vi "test read UDP low.vi"() -> ()   [LabVIEW 2019]
uses:
  Controls/UDP - Command.ctl
  Controls/UDP - Event.ctl
  Controls/UDP - Status.ctl
  Controls/Communication - Write Data.ctl
panel:
  in  "Datalog":T1(ring)
  out "Channels":T2
  in  "local port":u16=4001
  in  "Zero":T3(ring)
  in  "remote port":u16=4001
  in  "address":string="192.168.88.50"
  out "Data System":T4
  in  "Data":T5
  out "Data ADC":T6
  out "PID Setting":T7
  out "Sensor Out":T8
  out "Test SP":T9
  out "Status":T10 items=["Stop", "Ramp Up", "Ramp Down", "Jog Up", "Jog Down", "PID Mode", "PID Ramp"]
  out "Event":T11 items=["Stop", "Running", "PID", "Up Limit", "Down Limit", "Load Limit"]
  out "CMD Decimal Form":u8[](array[numeric])
  out "CMD HEX Form":string
  out "x+y":i32
  in  "CMD":T12
  out "data out":string
  out "Numeric 2":u8
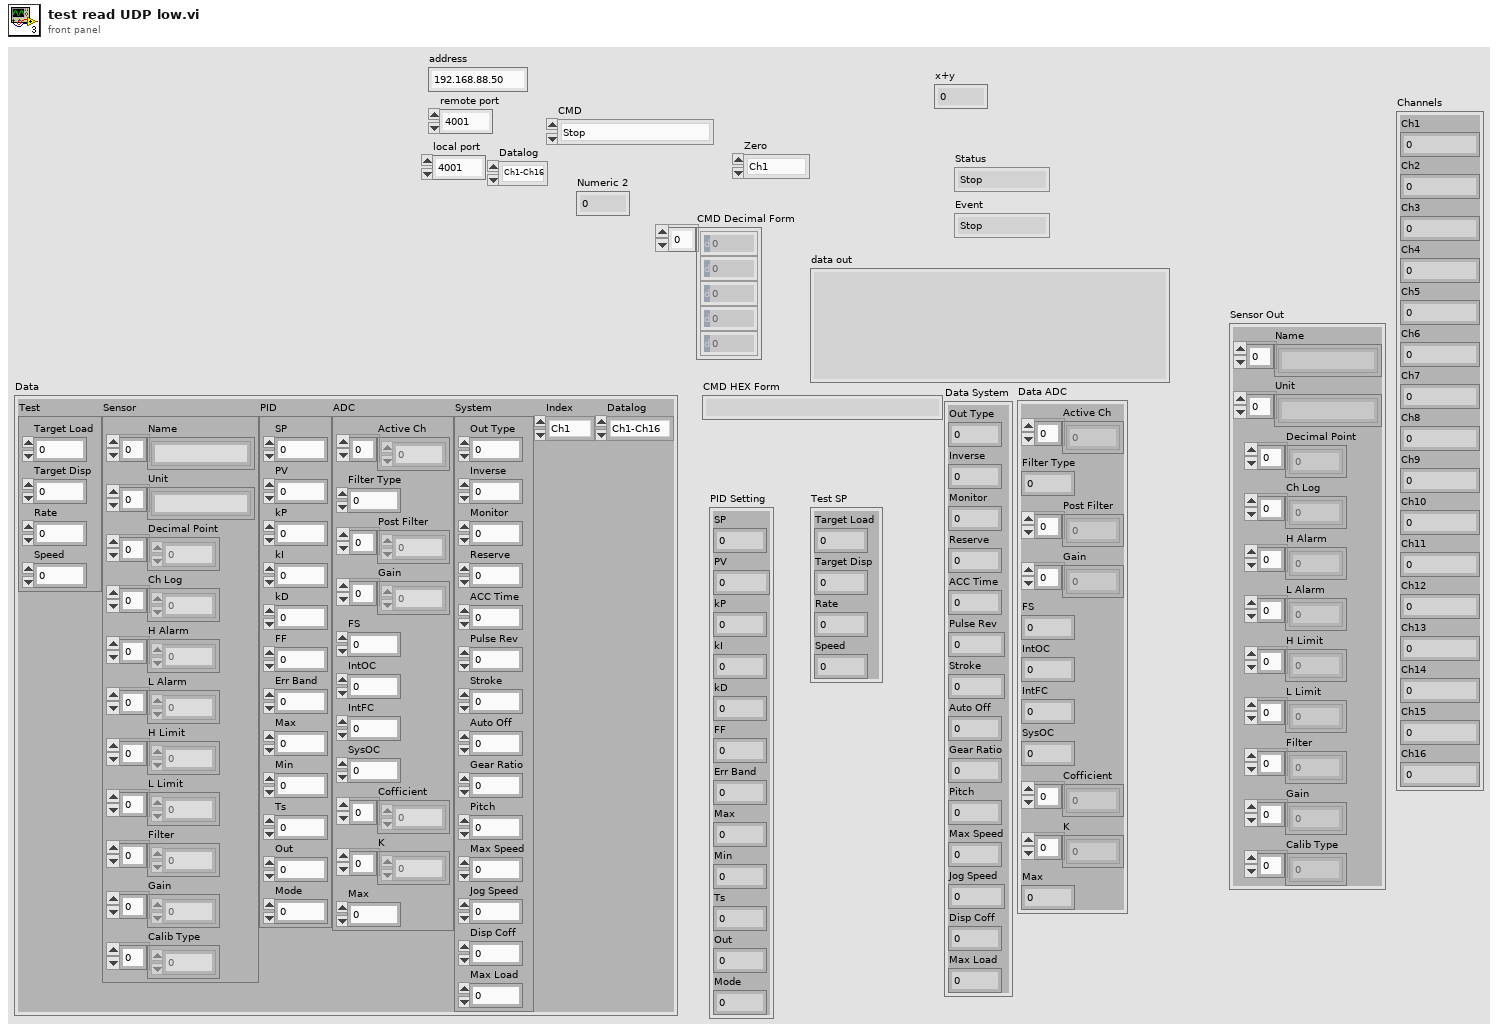
[diagram p1: front panel]
types:
  T1 = enum16{"Ch1-Ch16", "Ch17-Ch32", "Ch32-Ch48", "Ch49-Ch64", "Empty"}
  T2 = cluster{"Ch1":sgl, "Ch2":sgl, "Ch3":sgl, "Ch4":sgl, "Ch5":sgl, "Ch6":sgl, "Ch7":sgl, "Ch8":sgl, "Ch9":sgl, "Ch10":sgl, "Ch11":sgl, "Ch12":sgl, "Ch13":sgl, "Ch14":sgl, "Ch15":sgl, "Ch16":sgl}
  T3 = enum16{"Ch1", "Ch2", "Ch3", "Ch4", "Ch5", "Ch6", "Ch7", "Ch8", "Ch9", "Ch10", "Ch11", "Ch12", "Ch13", "Ch14", "Ch15", "Ch16"}
  T4 = cluster{"Out Type":u8, "Inverse":u8, "Monitor":u8, "Reserve":u8, "ACC Time":u32, "Pulse Rev":u32, "Stroke":u32, "Auto Off":u32, "Gear Ratio":sgl, "Pitch":sgl, "Max Speed":u32, "Jog Speed":u32, "Disp Coff":sgl, "Max Load":u32}
  T5 = typedef "Communication - Write Data.ctl" = cluster{"Test":cluster{"Target Load":sgl, "Target Disp":sgl, "Rate":sgl, "Speed":sgl}, "Sensor":cluster{"Name":string[], "Unit":string[], "Decimal Point":u8[], "Ch Log":u8[], "H Alarm":u8[], "L Alarm":u8[], "H Limit":sgl[], "L Limit":sgl[], "Filter":u8[], "Gain":u8[], "Calib Type":u32[]}, "PID":cluster{"SP":sgl, "PV":sgl, "kP":sgl, "kI":sgl, "kD":sgl, "FF":sgl, "Err Band":sgl, "Max":i32, "Min":i32, "Ts":u32, "Out":i32, "Mode":u8}, "ADC":cluster{"Active Ch":u8[], "Filter Type":u8, "Post Filter":u8[], "Gain":u8[], "FS":u16, "IntOC":u8, "IntFC":u8, "SysOC":u8, "Cofficient":dbl[], "K":dbl[], "Max":i32}, "System":cluster{"Out Type":u8, "Inverse":u8, "Monitor":u8, "Reserve":u8, "ACC Time":u32, "Pulse Rev":u32, "Stroke":u32, "Auto Off":u32, "Gear Ratio":sgl, "Pitch":sgl, "Max Speed":u32, "Jog Speed":u32, "Disp Coff":sgl, "Max Load":u32}, "Index":enum16{"Ch1", "Ch2", "Ch3", "Ch4", "Ch5", "Ch6", "Ch7", "Ch8", "Ch9", "Ch10", "Ch11", "Ch12", "Ch13", "Ch14", "Ch15", "Ch16"}, "Datalog":enum16{"Ch1-Ch16", "Ch17-Ch32", "Ch32-Ch48", "Ch49-Ch64", "Empty"}}
  T6 = cluster{"Active Ch":u8[], "Filter Type":u8, "Post Filter":u8[], "Gain":u8[], "FS":u16, "IntOC":u8, "IntFC":u8, "SysOC":u8, "Cofficient":dbl[], "K":dbl[], "Max":i32}
  T7 = cluster{"SP":sgl, "PV":sgl, "kP":sgl, "kI":sgl, "kD":sgl, "FF":sgl, "Err Band":sgl, "Max":i32, "Min":i32, "Ts":u32, "Out":i32, "Mode":u8}
  T8 = cluster{"Name":string[], "Unit":string[], "Decimal Point":u8[], "Ch Log":u8[], "H Alarm":u8[], "L Alarm":u8[], "H Limit":sgl[], "L Limit":sgl[], "Filter":u8[], "Gain":u8[], "Calib Type":u32[]}
  T9 = cluster{"Target Load":sgl, "Target Disp":sgl, "Rate":sgl, "Speed":sgl}
  T10 = typedef "UDP - Status.ctl" = u16
  T11 = typedef "UDP - Event.ctl" = u16
  T12 = typedef "UDP - Command.ctl" = enum16{"Stop", "Jog Up", "Jog Down", "Ramp Up", "Ramp Down", "PID Target", "PID Ramp", "Disp Run", "Read Ch Data", "Zero Channel", "Zero Disp", "Read Sensor", "Write Sensor", "Read ADC", "Write ADC", "Read PID", "Write PID", "Read Test", "Write Test", "Read System", "Write System", "Read Datalog", "Read Datalog Sensor"}
  T13 = cluster{"Target Load":sgl, "Target Disp":sgl, "Rate":sgl, "Ch4":sgl}
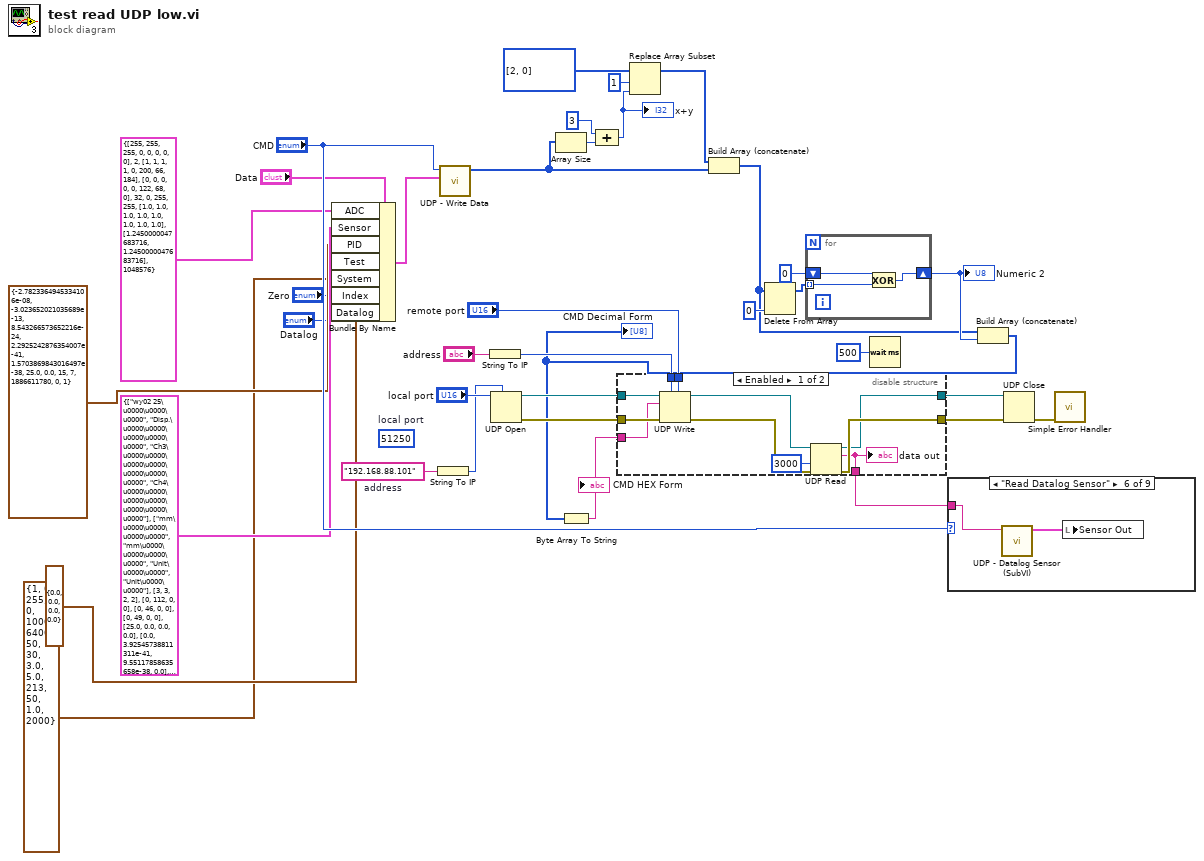
[diagram p0: block diagram]
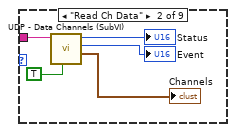
[diagram p4: hidden frame]
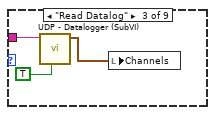
[diagram p5: hidden frame]
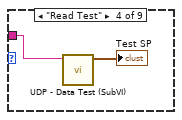
[diagram p6: hidden frame]
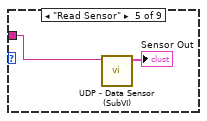
[diagram p7: hidden frame]
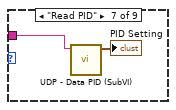
[diagram p8: hidden frame]
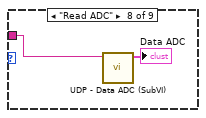
[diagram p9: hidden frame]
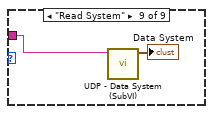
[diagram p10: hidden frame]
diagram:
  (unwired) u16 51250  # local port
  w4 = "192.168.88.101"  # address
  n1 = Bundle By Name(cluster="Data", "ADC"=T6 {"Active Ch"=[255, 255, 255, 0, 0, 0, 0, 0], "Filter Type"=2, "Post Filter"=[1, 1, 1, 1, 0, 200, 66, 184], "Gain"=[0, 0, 0, 0, 0, 122, 68, 0], "FS"=32, "IntOC"=0, "IntFC"=255, "SysOC"=255, "Cofficient"=[1.0, 1.0, 1.0, 1.0, 1.0, 1.0, 1.0, 1.0], "K"=[1.2450000047683716, 1.2450000047683716], "Max"=1048576} ("Data ADC"), "Sensor"=T8 {"Name"=["wy02 25\u0000\u0000\u0000", "Disp.\u0000\u0000\u0000\u0000\u0000", "Ch3\u0000\u0000\u0000\u0000\u0000\u0000\u0000", "Ch4\u0000\u0000\u0000\u0000\u0000\u0000\u0000"], "Unit"=["mm\u0000\u0000\u0000\u0000", "mm\u0000\u0000\u0000\u0000", "Unit\u0000\u0000", "Unit\u0000\u0000"], "Decimal Point"=[3, 3, 2, 2], "Ch Log"=[0, 112, 0, 0], "H Alarm"=[0, 46, 0, 0], "L Alarm"=[0, 49, 0, 0], "H Limit"=[25.0, 0.0, 0.0, 0.0], "L Limit"=[0.0, 3.92546e-41, 9.551179e-38, 0.0], "Filter"=[15, 1, 1, 1], "Gain"=[0, 0, 0, 0], "Calib Type"=[7, 2, 2, 2]} ("Sensor Out"), "PID"=T7 {"SP"=-2.7823365e-08, "PV"=-3.023652e-13, "kP"=8.5432666e-24, "kI"=2.29252e-41, "kD"=1.570387e-38, "FF"=25.0, "Err Band"=0.0, "Max"=15, "Min"=7, "Ts"=1886611780, "Out"=0, "Mode"=1} ("PID Setting"), "Test"=T9 {"Target Load"=0.0, "Target Disp"=0.0, "Rate"=0.0, "Speed"=0.0} ("Test SP"), "System"=T4 {"Out Type"=1, "Inverse"=0, "Monitor"=255, "Reserve"=0, "ACC Time"=1000, "Pulse Rev"=6400, "Stroke"=50, "Auto Off"=30, "Gear Ratio"=3.0, "Pitch"=5.0, "Max Speed"=213, "Jog Speed"=50, "Disp Coff"=1.0, "Max Load"=2000} ("Data System"), "Index"="Zero", "Datalog"="Datalog") -> (w9:T5)
  n2 = String To IP(1:w4) -> (0:w3:u32)
  n3 = call "UDP - Write Data.vi"("Data"=w9, "CMD"="CMD") -> ("Array"=w13:u8[])  [unwired: 9 in]
  n4 = String To IP(1:"address") -> (0:w35:u32)
  n5 = UDP Open(7:w3, 11:"local port") -> (port=w34:refnum<k16>, 0:w33:errorcluster)  [unwired: 3 in, 1 out]
  n6 = Array Size(array=w13) -> (size(s)=w19:i32)
  n7 = Compound Arithmetic op=ADD(3 ("x"), w19) -> (w17:i32)
  "x+y" <- w17
  n8 = Replace Array Subset(array=u8[] [2, 0], new element=w17, index=1) -> (w21:u8[])
  n9 = Build Array (concatenate)(w21, w13) -> (w20:u8[])
  n10 = Delete From Array(array=w20, index=0) -> (array with subset deleted=w27:u8[])  [unwired: 1 in, 1 out]
  n11 = for {
    shift-right: [w39] -> w26
    shift-left: u8 0 ("Numeric") -> [w40]
    tunnel: w27 -> [w38] mode=indexing
    n12 = Exclusive Or(1:w38, 2:w40) -> (0:w39:u8)
  }
  "Numeric 2" <- w26
  n13 = Wait (ms)(milliseconds to wait=u32 500) -> ()  [unwired: 1 out]
  n14 = Build Array (concatenate)(w20, w26) -> (w16:u8[])
  "CMD Decimal Form" <- w16
  n15 = Byte Array To String(unsigned byte array=w16) -> (string=w15:string)
  "CMD HEX Form" <- w15
  n16 = disable-structure shown="Enabled" {
    disable-tunnel: w35 -> [w51 _]
    disable-tunnel: w34 -> [w50 w54]
    disable-tunnel: w33 -> [w49 w53]
    disable-tunnel: "remote port" -> [w48 _]
    disable-tunnel: [w46 w53] -> w25
    disable-tunnel: [w44 w54] -> w24
    disable-tunnel: w15 -> [w43 w52]
    disable-tunnel: [w42 w52] -> w14
    frame Enabled {
      n17 = UDP Write(address=w51, port or service name=w48, connection ID=w50, data in=w43, 8:w49) -> (error out=w47:errorcluster, 3:w45:refnum<k16>)  [unwired: 1 in]
      n18 = UDP Read(connection ID=w45, timeout ms (25000)=3000, 8:w47) -> (data out=w42:string, error out=w46:errorcluster, 3:w44:refnum<k16>)  [unwired: 1 in, 2 out]
      "data out" <- w42
    }
    frame Disabled {
    }
  }
  n19 = case shown="\"Read Datalog Sensor\"" "CMD" {
    tunnel: w14 -> [_ w59 w62 w64 w66 w68 w70 w72 w74]
    frame "Stop", Default {
    }
    frame "Read Ch Data" {
      n20 = call "UDP - Data Channels (SubVI).vi"("test?"=TRUE, "data in"=w59) -> ("Channels"=→"Channels":T2, "Event"=→"Event":T11, "Status"=→"Status":T10)  [unwired: 5 in, 2 out]
    }
    frame "Read Datalog" {
      n21 = call "UDP - Datalogger (SubVI).vi"("test?"=TRUE, "data in"=w62) -> ("Channels"=w60:T2)  [unwired: 7 in, 2 out]
      n22 = local write "Channels"(w60) -> ()
    }
    frame "Read Test" {
      n23 = call "UDP - Data Test (SubVI).vi"("data in"=w64) -> ("Data Test"=→"Test SP":T13)  [unwired: 8 in, 2 out]
    }
    frame "Read Sensor" {
      n24 = call "UDP - Data Sensor (SubVI).vi"("String"=w66) -> ("Sensor Out"=→"Sensor Out":T8)  [unwired: 8 in, 2 out]
    }
    frame "Read Datalog Sensor" {
      n25 = call "UDP - Datalog Sensor (SubVI).vi"("String"=w68) -> ("Sensor Out"=w67:T8)  [unwired: 8 in, 2 out]
      n26 = local write "Sensor Out"(w67) -> ()
    }
    frame "Read PID" {
      n27 = call "UDP - Data PID (SubVI).vi"("Data"=w70) -> ("PID Setting"=→"PID Setting":T7)  [unwired: 8 in, 2 out]
    }
    frame "Read ADC" {
      n28 = call "UDP - Data ADC (SubVI).vi"("Data"=w72) -> ("Data ADC"=→"Data ADC":T6)  [unwired: 8 in, 2 out]
    }
    frame "Read System" {
      n29 = call "UDP - Data System (SubVI).vi"("Data"=w74) -> ("Data System"=→"Data System":T4)  [unwired: 8 in, 2 out]
    }
  }
  n30 = UDP Close(connection ID=w24, 8:w25) -> (error out=w36:errorcluster)  [unwired: 1 out]
  n31 = call <vilib>:"Simple Error Handler.vi"("error in (no error)"=w36) -> ()  [unwired: 4 in, 5 out]
